vi "main.vi"() -> ()   [LabVIEW 2020]
uses:
  <vilib>/express/express arith-compare/Formula/XNode/ExpressFormulaBlockNode.xnode
  <vilib>/measure/NI_MABase.lvlib
  <vilib>/Analysis/NI_AALPro.lvlib
panel:
  out "采样率 Hz 4":dbl
  out "采样数 4":dbl
  out "采样数 3":dbl
  out "采样率 Hz 3":dbl
  out "采样数":dbl
  out "采样率 Hz":dbl
  out "采样率/采样数":dbl
  in  "Tab Control":enum32{"余弦信号", "余弦信号叠加", "数字基带信号", "三阶 m 序列"}(tab)
  in  "k_f kHz/V":dbl=50.0
  in  "A_c V":dbl=1.0
  in  "f_c kHz":dbl=150.0
  in  "采样率 MHz":dbl=50.0
  in  "Lower Cut-Off Hz":dbl=280000.0 caption="Lower Cut-Off"
  in  "标准差 V":dbl=0.02 format="%.2p"
  in  "采样数 k":dbl=3000.0
  in  "A_m V":dbl=1.0
  in  "f_m kHz":dbl=5.0
  in  "Useless":enum32{"时域特性", "频域特性"}(tab)
  out "信号时域波形观测":dynamicdata(graph)
  out "解调复原的基带信号":waveform(dbl)(graph)
  out "已调信号频域波形观测":dynamicdata(graph)
  out "实测已调信号带宽 Hz":dbl
  out "理论已调信号带宽 Hz":dbl
  in  "Tab Control 2":enum32{"时域特性", "频域特性"}(tab)
  out "信号时域波形观测":dynamicdata(graph)
  out "解调复原的基带信号":waveform(dbl)(graph)
  out "已调信号频域波形观测":dynamicdata(graph)
  in  "f_m1 kHz":dbl=5.0
  in  "A_m1 V":dbl=1.0
  in  "采样数 k":dbl=3000.0
  in  "标准差 V":dbl=0.1 format="%.2p"
  in  "Lower Cut-Off Hz":dbl=330000.0 caption="Lower Cut-Off"
  in  "采样率 MHz":dbl=50.0
  in  "f_c kHz":dbl=150.0
  in  "A_c V":dbl=1.0
  in  "k_f kHz/V":dbl=50.0
  in  "f_m2 kHz":dbl=3.0
  in  "A_m2 V":dbl=1.0
  out "采样率 Hz 2":dbl
  out "采样数 2":dbl
  in  "Useless 2":enum32{"时域特性", "频域特性"}(tab)
  out "信号时域波形观测":dynamicdata(graph)
  out "解调复原的基带信号":waveform(dbl)(graph)
  out "已调信号频域波形观测":dynamicdata(graph)
  in  "T us":dbl=200.0
  in  "A_m V":dbl=1.0
  in  "采样数 k":dbl=3000.0
  in  "标准差 V":dbl=0.1 format="%.2p"
  in  "Lower Cut-Off Hz":dbl=280000.0 caption="Lower Cut-Off"
  in  "采样率 MHz":dbl=50.0
  in  "f_c kHz":dbl=150.0
  in  "A_c V":dbl=1.0
  in  "k_f kHz/V":dbl=50.0
  in  "k_f kHz/V":dbl=50.0
  in  "A_c V":dbl=1.0
  in  "f_c kHz":dbl=150.0
  in  "采样率 MHz":dbl=50.0
  in  "Lower Cut-Off Hz":dbl=280000.0 caption="Lower Cut-Off"
  in  "标准差 V":dbl=0.1 format="%.2p"
  in  "采样数 k":dbl=3000.0
  in  "A_m V":dbl=1.0
  in  "T us":dbl=200.0
  in  "Useless 3":enum32{"时域特性", "频域特性"}(tab)
  out "信号时域波形观测":dynamicdata(graph)
  out "解调复原的基带信号":waveform(dbl)(graph)
  out "已调信号频域波形观测":dynamicdata(graph)
  # "调制信号工作参数"
  # "载波信号工作参数"
  # "调制参数"
  # "解调参数"
  # "仿真参数"
  # "调制信号工作参数"
  # "载波信号工作参数"
  # "调制参数"
  # "解调参数"
  # "仿真参数"
  # "调制信号工作参数"
  # "载波信号工作参数"
  # "调制参数"
  # "解调参数"
  # "仿真参数"
  # "调制信号工作参数"
  # "载波信号工作参数"
  # "调制参数"
  # "解调参数"
  # "仿真参数"
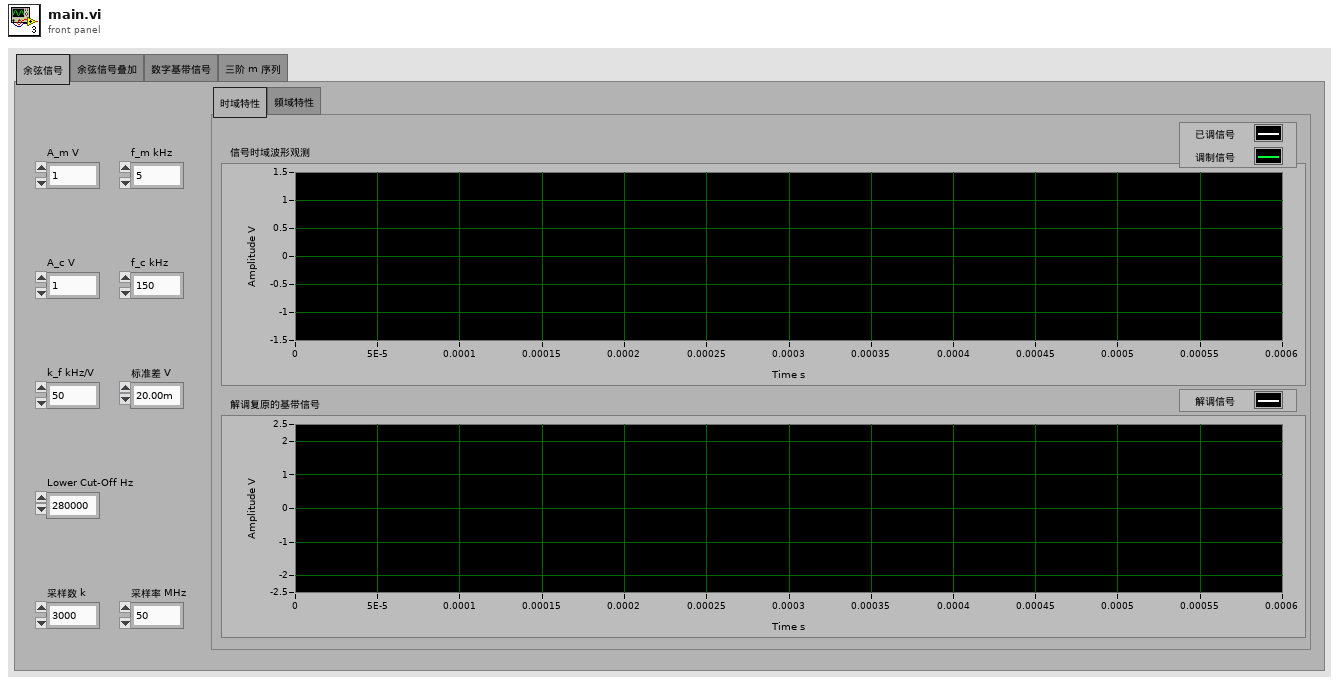
[diagram p1: front panel]
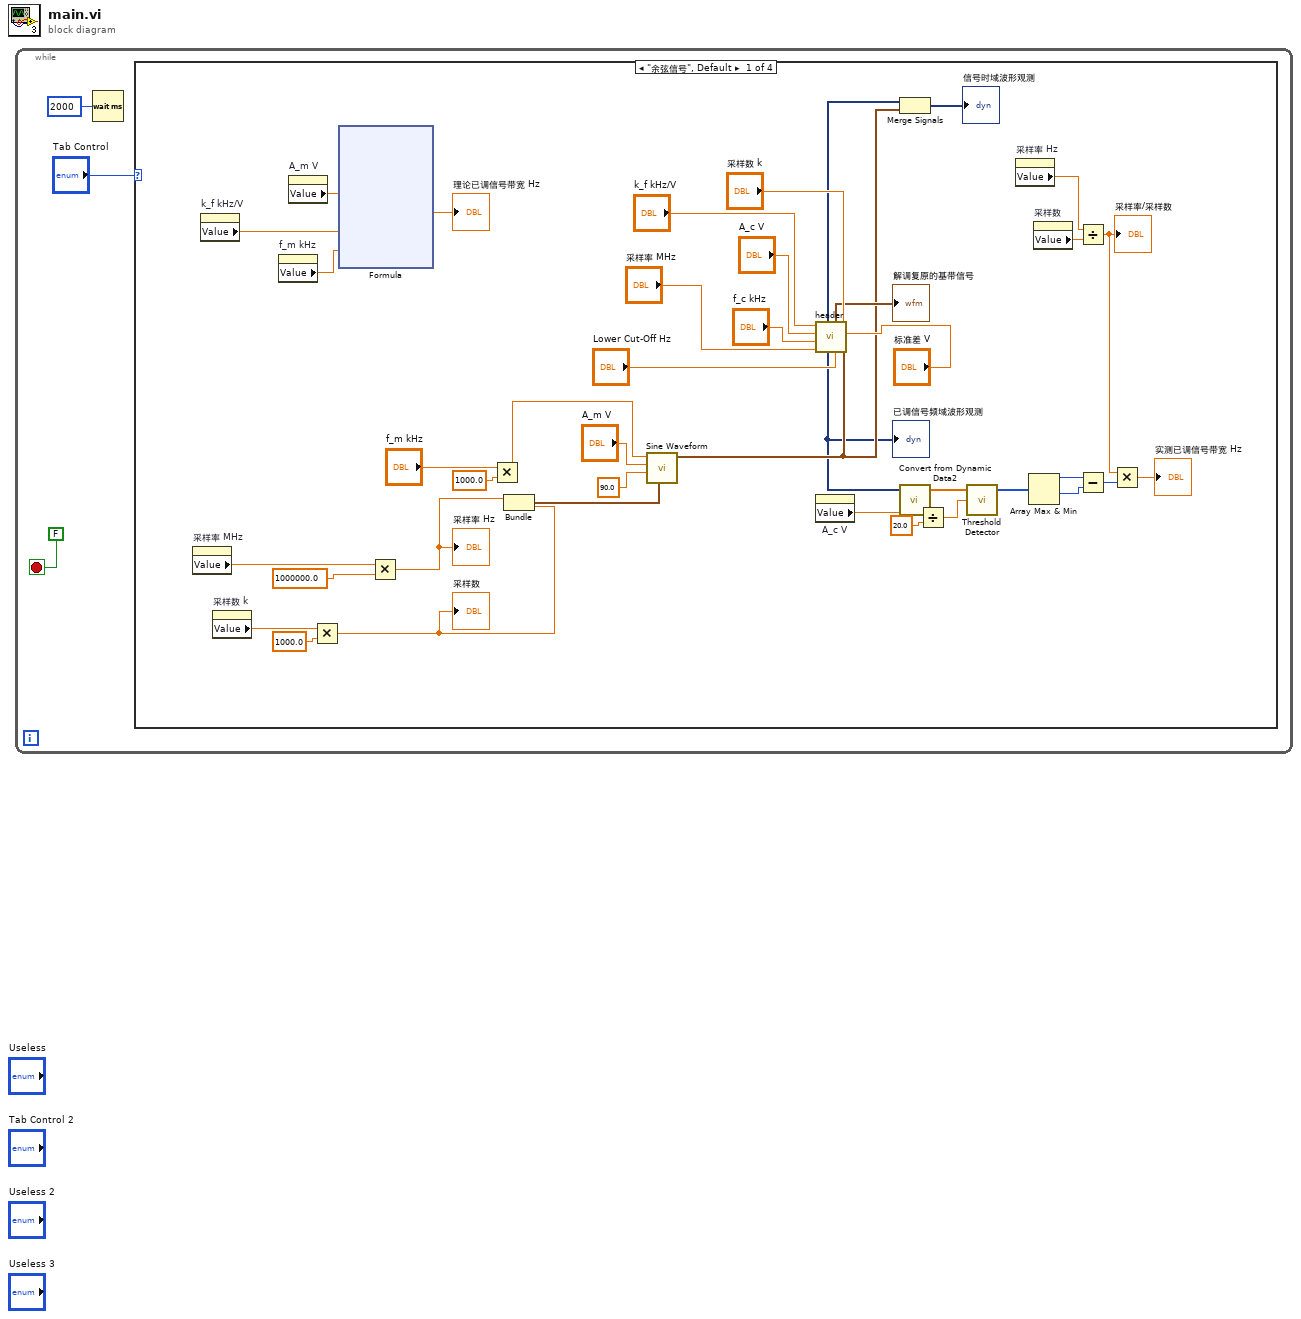
[diagram p0: block diagram]
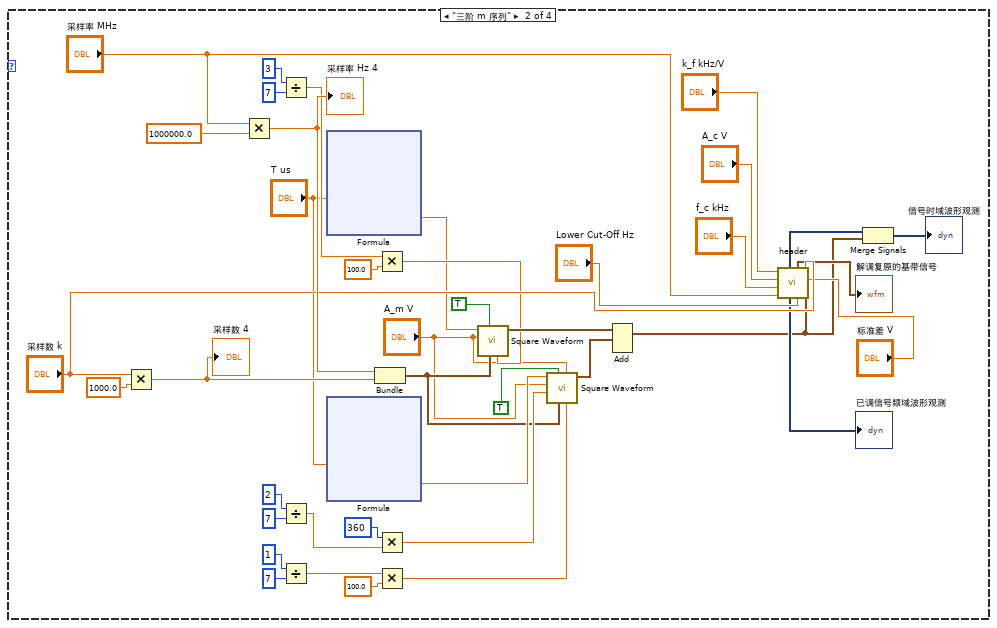
[diagram p2: hidden frame]
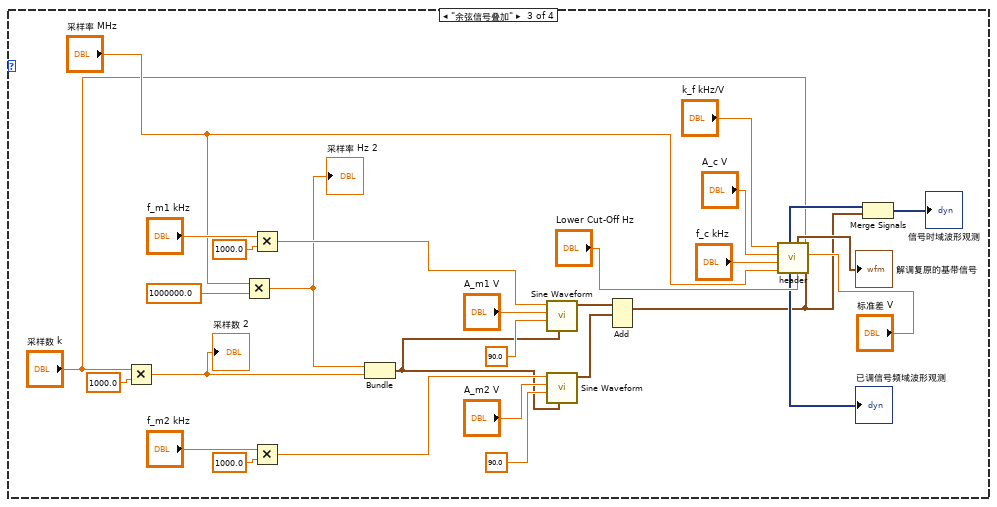
[diagram p3: hidden frame]
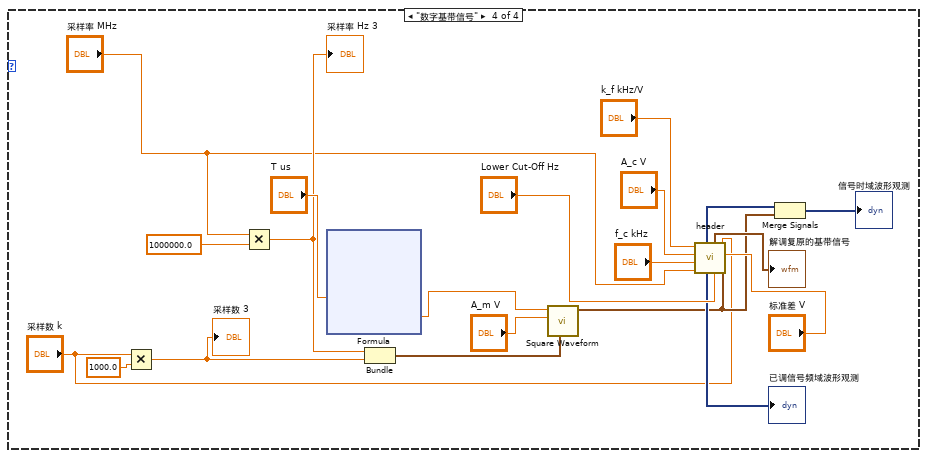
[diagram p4: hidden frame]
diagram:
  n1 = while {
    stop <- FALSE stop-if-true
    n2 = Wait (ms)(milliseconds to wait=u32 2000) -> ()  [unwired: 1 out]
    n3 = case shown="\"余弦信号\", Default" "Tab Control" {
      frame "余弦信号", Default {
        n4 = property on="采样率 MHz" class="DigNum (strict)"() -> ("Value"=w8:dbl)  [unwired: 2 in, 2 out]
        n5 = property on="k_f kHz/V" class="DigNum (strict)"() -> ("Value"=w10:dbl)  [unwired: 2 in, 2 out]
        n6 = property on="采样数 k" class="DigNum (strict)"() -> ("Value"=w7:dbl)  [unwired: 2 in, 2 out]
        n7 = property on="f_m kHz" class="DigNum (strict)"() -> ("Value"=w9:dbl)  [unwired: 2 in, 2 out]
        n8 = property on="A_m V" class="DigNum (strict)"() -> ("Value"=w11:dbl)  [unwired: 2 in, 2 out]
        n9 = Multiply(x=w7, y=1000.0) -> (x*y=w17:dbl)
        "采样数" <- w17
        n10 = xnode "Formula"("A_m"=w11, "k_f"=w10, "F_m"=w9) -> ("Result"=→"理论已调信号带宽 Hz":dbl)  [unwired: 1 in, 1 out]
        n11 = Multiply(x=w8, y=1000000.0) -> (x*y=w19:dbl)
        "采样率 Hz" <- w19
        n12 = Multiply(x="f_m kHz", y=1000.0) -> (x*y=w21:dbl)
        n13 = Bundle(w19, w17) -> (w16:cluster{dbl, dbl})  [unwired: 1 in]
        n14 = call <vilib>:"Sine Waveform.vi"("sampling info"=w16, "phase"=90.0, "amplitude"="A_m V", "frequency"=w21) -> ("signal out"=w15:waveform(dbl))  [unwired: 6 in, 1 out]
        n15 = call "header.vi"("Signals"=w15, "标准差 V"="标准差 V", "采样数 k"="采样数 k", "Lower Cut-Off"="Lower Cut-Off Hz", "采样率 MHz"="采样率 MHz", "f_c kHz"="f_c kHz", "A_c V"="A_c V", "k_f kHz/V"="k_f kHz/V") -> ("解调复原的基带信号"=→"解调复原的基带信号":waveform(dbl), "已调信号频域波形观测"=w14:dynamicdata, "信号时域波形观测"=w26:dynamicdata)  [unwired: 1 in]
        "已调信号频域波形观测" <- w14
        n16 = property on="A_c V" class="DigNum (strict)"() -> ("Value"=w6:dbl)  [unwired: 2 in, 2 out]
        n17 = Merge Signals(w26, w15) -> (→"信号时域波形观测":dynamicdata)
        n18 = call "Convert from Dynamic Data2"("Dynamic Data Type"=w14) -> ("Array"=w43:dbl[])  [unwired: 3 in]
        n19 = Divide(x=w6, y=20.0) -> (x/y=w4:dbl)
        n20 = call <vilib>:"Threshold Detector.vi"("threshold"=w4, "X"=w43) -> ("Indices"=w37:i32[])  [unwired: 1 in, 2 out]
        n21 = property on="采样率 Hz" class="DigNum (strict)"() -> ("Value"=w12:dbl)  [unwired: 2 in, 2 out]
        n22 = Array Max & Min(array=w37) -> (max value=w42:i32, min value=w41:i32)  [unwired: 2 out]
        n23 = property on="采样数" class="DigNum (strict)"() -> ("Value"=w13:dbl)  [unwired: 2 in, 2 out]
        n24 = Divide(x=w12, y=w13) -> (x/y=w39:dbl)
        "采样率/采样数" <- w39
        n25 = Subtract(x=w42, y=w41) -> (x-y=w40:i32)
        n26 = Multiply(x=w39, y=w40) -> (x*y=→"实测已调信号带宽 Hz":dbl)
      }
      frame "三阶 m 序列" {
        n27 = Multiply(x="采样数 k", y=1000.0) -> (x*y=w91:dbl)
        "采样数 4" <- w91
        n28 = Multiply(x="采样率 MHz", y=1000000.0) -> (x*y=w93:dbl)
        "采样率 Hz 4" <- w93
        n29 = Divide(x=3, y=7) -> (x/y=w73:dbl)
        n30 = Divide(x=2, y=7) -> (x/y=w77:dbl)
        n31 = Divide(x=1, y=7) -> (x/y=w75:dbl)
        n32 = xnode "Formula"("T"="T us") -> ("Result"=w71:dbl)  [unwired: 1 in, 1 out]
        n33 = xnode "Formula"("T"="T us") -> ("Result"=w72:dbl)  [unwired: 1 in, 1 out]
        n34 = Bundle(w93, w91) -> (w61:cluster{dbl, dbl})  [unwired: 1 in]
        n35 = Multiply(x=w73, y=100.0) -> (x*y=w74:dbl)
        n36 = Multiply(x=360, y=w77) -> (x*y=w78:dbl)
        n37 = Multiply(x=w75, y=100.0) -> (x*y=w76:dbl)
        n38 = call <vilib>:"Square Waveform.vi"("duty cycle (%)"=w74, "sampling info"=w61, "reset signal"=TRUE, "amplitude"="A_m V", "frequency"=w71) -> ("signal out"=w80:waveform(dbl))  [unwired: 5 in, 1 out]
        n39 = call <vilib>:"Square Waveform.vi"("duty cycle (%)"=w76, "offset"="A_m V", "sampling info"=w61, "reset signal"=TRUE, "phase"=w78, "amplitude"="A_m V", "frequency"=w72) -> ("signal out"=w79:waveform(dbl))  [unwired: 3 in, 1 out]
        n40 = Add(1:w79, 2:w80) -> (0:w58:waveform(dbl))  [unwired: 1 in, 1 out]
        n41 = call "header.vi"("Signals"=w58, "标准差 V"="标准差 V", "采样数 k"="采样数 k", "Lower Cut-Off"="Lower Cut-Off Hz", "采样率 MHz"="采样率 MHz", "f_c kHz"="f_c kHz", "A_c V"="A_c V", "k_f kHz/V"="k_f kHz/V") -> ("解调复原的基带信号"=→"解调复原的基带信号":waveform(dbl), "已调信号频域波形观测"=→"已调信号频域波形观测":dynamicdata, "信号时域波形观测"=w95:dynamicdata)  [unwired: 1 in]
        n42 = Merge Signals(w95, w58) -> (→"信号时域波形观测":dynamicdata)
      }
      frame "余弦信号叠加" {
        n43 = Multiply(x="采样数 k", y=1000.0) -> (x*y=w116:dbl)
        "采样数 2" <- w116
        n44 = Multiply(x="采样率 MHz", y=1000000.0) -> (x*y=w118:dbl)
        "采样率 Hz 2" <- w118
        n45 = Multiply(x="f_m1 kHz", y=1000.0) -> (x*y=w129:dbl)
        n46 = Multiply(x="f_m2 kHz", y=1000.0) -> (x*y=w128:dbl)
        n47 = Bundle(w118, w116) -> (w113:cluster{dbl, dbl})  [unwired: 1 in]
        n48 = call <vilib>:"Sine Waveform.vi"("sampling info"=w113, "phase"=90.0, "amplitude"="A_m1 V", "frequency"=w129) -> ("signal out"=w125:waveform(dbl))  [unwired: 6 in, 1 out]
        n49 = call <vilib>:"Sine Waveform.vi"("sampling info"=w113, "phase"=90.0, "amplitude"="A_m2 V", "frequency"=w128) -> ("signal out"=w124:waveform(dbl))  [unwired: 6 in, 1 out]
        n50 = Add(1:w124, 2:w125) -> (0:w112:waveform(dbl))  [unwired: 1 in, 1 out]
        n51 = call "header.vi"("Signals"=w112, "标准差 V"="标准差 V", "采样数 k"="采样数 k", "Lower Cut-Off"="Lower Cut-Off Hz", "采样率 MHz"="采样率 MHz", "f_c kHz"="f_c kHz", "A_c V"="A_c V", "k_f kHz/V"="k_f kHz/V") -> ("解调复原的基带信号"=→"解调复原的基带信号":waveform(dbl), "已调信号频域波形观测"=→"已调信号频域波形观测":dynamicdata, "信号时域波形观测"=w132:dynamicdata)  [unwired: 1 in]
        n52 = Merge Signals(w132, w112) -> (→"信号时域波形观测":dynamicdata)
      }
      frame "数字基带信号" {
        n53 = Multiply(x="采样数 k", y=1000.0) -> (x*y=w144:dbl)
        "采样数 3" <- w144
        n54 = Multiply(x="采样率 MHz", y=1000000.0) -> (x*y=w146:dbl)
        "采样率 Hz 3" <- w146
        n55 = xnode "Formula"("T"="T us") -> ("Result"=w151:dbl)  [unwired: 1 in, 1 out]
        n56 = Bundle(w146, w144) -> (w141:cluster{dbl, dbl})  [unwired: 1 in]
        n57 = call <vilib>:"Square Waveform.vi"("sampling info"=w141, "amplitude"="A_m V", "frequency"=w151) -> ("signal out"=w148:waveform(dbl))  [unwired: 7 in, 1 out]
        n58 = call "header.vi"("Signals"=w148, "标准差 V"="标准差 V", "采样数 k"="采样数 k", "Lower Cut-Off"="Lower Cut-Off Hz", "采样率 MHz"="采样率 MHz", "f_c kHz"="f_c kHz", "A_c V"="A_c V", "k_f kHz/V"="k_f kHz/V") -> ("解调复原的基带信号"=→"解调复原的基带信号":waveform(dbl), "已调信号频域波形观测"=→"已调信号频域波形观测":dynamicdata, "信号时域波形观测"=w152:dynamicdata)  [unwired: 1 in]
        n59 = Merge Signals(w152, w148) -> (→"信号时域波形观测":dynamicdata)
      }
    }
  }
